vi "CAN Name Search Unit.vi"(11 "Gas Name":T1) -> (0 "Min":dbl, 1 "Max":dbl, 2 "Unit":string, 3 "Gefunden?":bool)   [LabVIEW 2020, in "CAN Konfig.lvlib"]
uses:
  CAN Konfig.lvlib
  Visualisierungs Elemente/String - Ausgabefeld.ctl
  Gaszuordnung AO/FGV Gaszuordnung Grenzen&Einheit Aktion.ctl
  Gaszuordnung AO/Gaszuordnung AO.lvlib
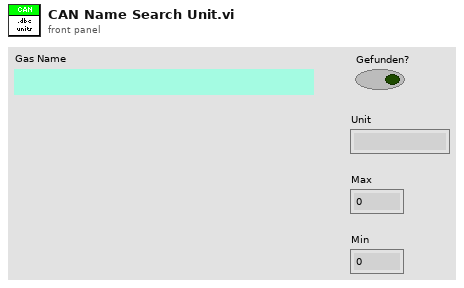
[diagram p1: front panel]
types:
  T1 = typedef "String - Ausgabefeld.ctl" = string
  T2 = typedef "Gaszuordnung AO.lvlib/FGV Gaszuordnung Grenzen&Einheit Aktion.ctl" = enum16{"Lesen", "Schreiben Min", "Schreiben Max", "Laden", "Speichern"}
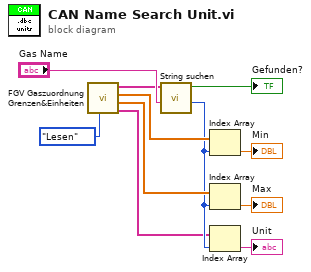
[diagram p0: block diagram]
diagram:
  n1 = call "FGV Gaszuordnung Grenzen&Einheiten.vi"("Aktion"=FGV_Gaszuordnung_Grenzen&Einheit_Aktion."Lesen") -> ("Einheit neu"=w3:string[], "Max neu"=w6:dbl[], "Min neu"=w5:dbl[], "Namen neu"=w2:string[])  [unwired: 2 in, 5 out]
  n2 = call "String suchen.vi"("Gasname"="Gas Name", "Such-Namen"=w2) -> ("Index"=w4:i32, "Gefunden?"=→"Gefunden?":bool)  [unwired: 8 in]
  n3 = Index Array(array=w5, index=w4) -> (element=→"Min":dbl)
  n4 = Index Array(array=w6, index=w4) -> (element=→"Max":dbl)
  n5 = Index Array(array=w3, index=w4) -> (element=→"Unit":string)
